vi "Gen - VI Transparency.vi"(6 "State":T1(ring)=enum."Standard", 8 "Error In":errorcluster, 9 "Transparency":u8, 10 "Transparently?":bool=TRUE, 11 "Ref VI":refnum<vi>) -> (0 "Error Out":errorcluster, 3 "Ref VI Out":refnum<vi>)   [LabVIEW 2020]
doc: "This VI use to set the Front Panel Transparency."
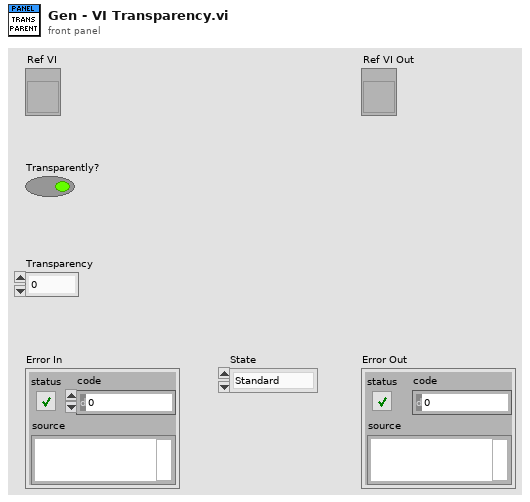
[diagram p1: front panel]
types:
  T1 = enum32{"Invalid", "Standard", "Closed", "Hidden", "Minimized", "Maximized"}
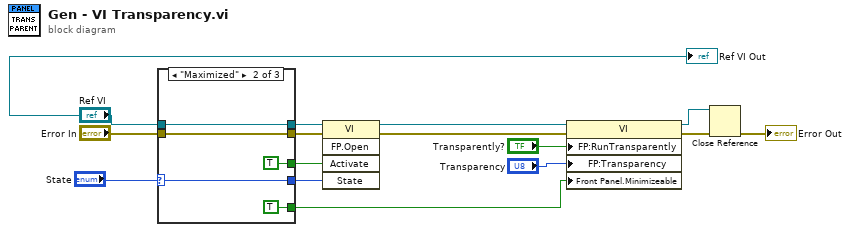
[diagram p0: block diagram]
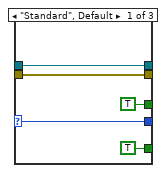
[diagram p2: hidden frame]
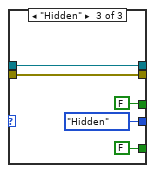
[diagram p3: hidden frame]
diagram:
  n1 = case shown="\"Maximized\"" "State" {
    selector: "State" -> [w16 w21 _]
    tunnel: [w16 w21 T1."Hidden" ("State")] -> w9
    tunnel: [TRUE ("Activate?") TRUE ("Activate?") FALSE ("Activate?")] -> w8
    tunnel: [w20 w25 w30] -> w14
    tunnel: "Error In" -> [w20 w25 w30]
    tunnel: [w18 w23 w27] -> w6
    tunnel: "Ref VI" -> [w18 w23 w27]
    tunnel: [TRUE ("Activate?") TRUE ("Activate?") FALSE ("Activate?")] -> w2
    frame "Standard", Default {
    }
    frame "Maximized" {
    }
    frame "Hidden" {
    }
  }
  n2 = invoke class="VI" method="FP.Open"(reference=w6, error in=w14, "Activate"=w8, "State"=w9) -> (reference out=w3:refnum<vi>, error out=w11:errorcluster)  [unwired: 1 in, 3 out]
  n3 = property class="VI"(reference=w3, error in=w11, "FP:RunTransparently"="Transparently?", "FP:Transparency"="Transparency", "Front Panel.Minimizeable"=w2) -> (reference out=w5:refnum<vi>, error out=w13:errorcluster)
  n4 = Close Reference(reference=w5, error in (no error)=w13) -> (error out=→"Error Out":errorcluster)
  "Ref VI Out" <- "Ref VI"
